vi "Format Time Stamp to XML dateTime string.vi"(8 "error in (no error)":errorcluster, 10 "time stamp":timestamp) -> (0 "error out":errorcluster, 2 "xml dateTime string":string)   [LabVIEW 2013]
panel:
  # "Copyright © 2008 James Kring, Inc. All rights reserved.\n\nAuthor: Jim Kring <jim.kring@jameskring.com>\n\nThis library is provided \"AS IS\" , WITHOUT WARRANTIES OR \nCONDITIONS OF ANY KIND, either express or implied.\n\nJames Kring, Inc. -- http://www.jameskring.com"
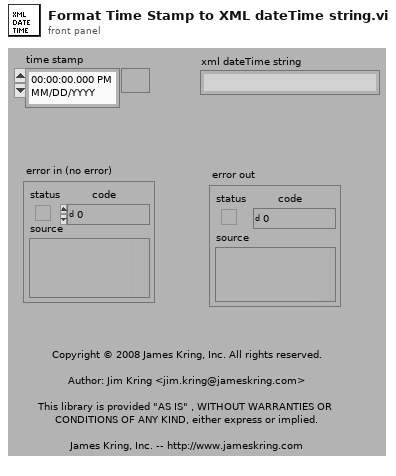
[diagram p1: front panel]
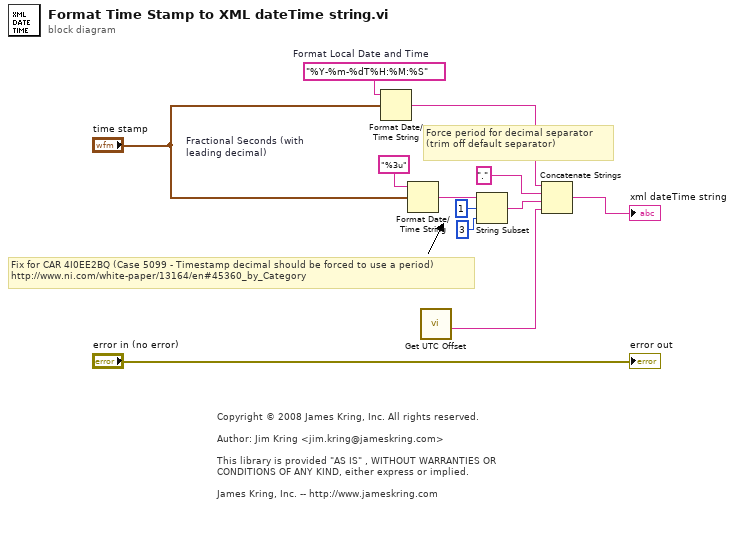
[diagram p0: block diagram]
diagram:
  w7 = "%3u"  # Fractional Seconds (with leading decimal)
  w10 = "%Y-%m-%dT%H:%M:%S"  # Format Local Date and Time
  # "Force period for decimal separator\n(trim off default separator)"
  # "Fix for CAR 4I0EE2BQ (Case 5099 - Timestamp decimal should be forced to use a period)\nhttp://www.ni.com/white-paper/13164/en#45360_by_Category"
  # "Copyright © 2008 James Kring, Inc. All rights reserved.\n\nAuthor: Jim Kring <jim.kring@jameskring.com>\n\nThis library is provided \"AS IS\" , WITHOUT WARRANTIES OR \nCONDITIONS OF ANY KIND, either express or implied.\n\nJames Kring, Inc. -- http://www.jameskring.com"
  n1 = Format Date/Time String(time format string (%c)=w10, seconds (now)="time stamp") -> (date/time string=w8:string)  [unwired: 1 in]
  n2 = Format Date/Time String(time format string (%c)=w7, seconds (now)="time stamp") -> (date/time string=w4:string)  [unwired: 1 in]
  n3 = call "Get UTC Offset.vi"() -> ("UTC Offset String"=w11:string)  [unwired: 10 in, 1 out]
  n4 = String Subset(string=w4, offset (0)=1, length (rest)=3 ("length (rest)")) -> (substring=w1:string)
  n5 = Concatenate Strings(w8, ".", w1, w11) -> (→"xml dateTime string":string)
  "error out" <- "error in (no error)"
